vi "TEST1.vi"() -> ()   [LabVIEW 2013]
panel:
  out "data":dynamicdata(graph) caption="données"
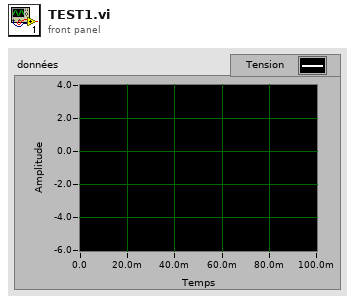
[diagram p1: front panel]
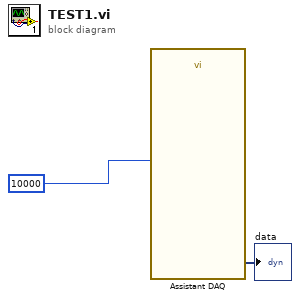
[diagram p0: block diagram]
diagram:
  n1 = call "Assistant DAQ"("vitesse"=10000) -> ("data"=→"data":dynamicdata)  [unwired: 16 in, 2 out]
